vi "Set Z Value Write.vi"(4 "error in (no error)":errorcluster, 5 "Value":dbl, 6 "Container State":T6, 7 "Display State In":T1={"Initialization"=TRUE, "Show in and out values"=TRUE, "Show Highliting"=TRUE, "Open Plot"=FALSE, "Format String"="%10_4g", "X"=0.0, "Y"=0.0, "Limits"={"Min X"=inf, "Max X"=inf, "MaxDiff X"=inf, "MaxGrad X"=inf, "Min Y"=inf, "Max Y"=inf, "MaxDiff Y"=inf, "MaxGrad Y"=inf, "Min Z"=inf, "Max Z"=inf, "MaxDiff Z"=inf}, "Vertical Scrollbar"=FALSE, "Horizontal Scrollbar"=FALSE, "Data"={"X"=[1.0, 2.0], "Y"=[3.0, 4.0], "Z"=[[5.0, 7.0], [6.0, 8.0]]}, "Undo Avaliable"=FALSE, "Root"=refnum, "Z"=0.0, "Links"=[], "Control Error"={"status"=FALSE, "code"=0, "source"=""}}) -> (0 "error out":errorcluster, 3 "Display State Out":T1={"Initialization"=TRUE, "Show in and out values"=TRUE, "Show Highliting"=TRUE, "Open Plot"=FALSE, "Format String"="%10_4g", "X"=0.0, "Y"=0.0, "Limits"={"Min X"=inf, "Max X"=inf, "MaxDiff X"=inf, "MaxGrad X"=inf, "Min Y"=inf, "Max Y"=inf, "MaxDiff Y"=inf, "MaxGrad Y"=inf, "Min Z"=inf, "Max Z"=inf, "MaxDiff Z"=inf}, "Vertical Scrollbar"=FALSE, "Horizontal Scrollbar"=FALSE, "Data"={"X"=[1.0, 2.0], "Y"=[3.0, 4.0], "Z"=[[5.0, 7.0], [6.0, 8.0]]}, "Undo Avaliable"=FALSE, "Root"=refnum, "Z"=0.0, "Links"=[], "Control Error"={"status"=FALSE, "code"=0, "source"=""}})   [LabVIEW 2011, in "XCPCCP TBL2D.xctl"]
uses:
  XCPCCP TBL2D.xctl
  <vilib>/_xctls/Container State.ctl
  State TBL2D.ctl
  Limits TBL2D.ctl
  Data TBL2D.ctl
  NationalInstruments.VeriStand.SystemStorage
  Controls/Control Links.ctl
  Controls/ECUMC Item.ctl
  <vilib>/_xctls/XControlSupport.lvlib
panel:
  # "Replace the Value Control below with a Control of desired type.\nDo not remove this Control or the others from the connector pane.\nDo not change the connector pane pattern.\nThe Value control should always be the third terminal from top on the input side in the connector pane."
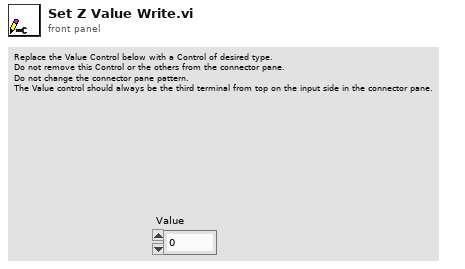
[diagram p1: front panel]
types:
  T1 = typedef "XCPCCP TBL2D.xctl/State TBL2D.ctl" = cluster{"Initialization":bool, "Show in and out values":bool, "Show Highliting":bool, "Open Plot":bool, "Format String":string, "X":sgl, "Y":sgl, "Limits":T2, "Vertical Scrollbar":bool, "Horizontal Scrollbar":bool, "Data":T3, "Undo Avaliable":bool, "Root":refnum<k24>, "Z":sgl, "Links":T4, "Control Error":errorcluster}
  T2 = typedef "XCPCCP TBL2D.xctl/Limits TBL2D.ctl" = cluster{"Min X":sgl, "Max X":sgl, "MaxDiff X":sgl, "MaxGrad X":sgl, "Min Y":sgl, "Max Y":sgl, "MaxDiff Y":sgl, "MaxGrad Y":sgl, "Min Z":sgl, "Max Z":sgl, "MaxDiff Z":sgl}
  T3 = typedef "XCPCCP TBL2D.xctl/Data TBL2D.ctl" = cluster{"X":sgl[], "Y":sgl[], "Z":sgl[][]}
  T4 = typedef "Control Links.ctl" = T5[]
  T5 = typedef "ECUMC Item.ctl" = cluster{"NodePath":string, "NodePathArray":string[]}
  T6 = typedef "XControlSupport.lvlib/Container State.ctl" = cluster{"Indicator?":bool, "Run Mode?":bool, " Refnum":refnum<vi>}
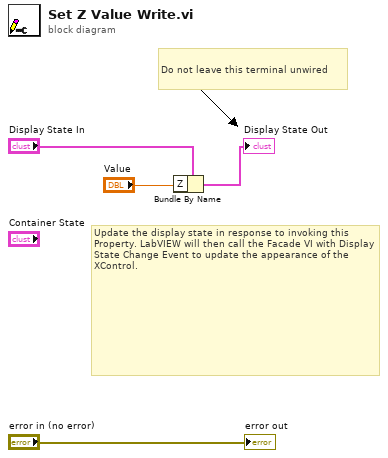
[diagram p0: block diagram]
diagram:
  # "Do not leave this terminal unwired"
  # "Update the display state in response to invoking this Property. LabVIEW will then call the Facade VI with Display State Change Event to update the appearance of the XControl."
  n1 = Bundle By Name(cluster="Display State In", "Z"="Value") -> (→"Display State Out":T1)
  "error out" <- "error in (no error)"
